vi "list and create PG table 64.vi"(6 "columns type (real)":string="real", 8 "error in":errorcluster, 9 "columns":string[](array[string]), 10 "table name":string, 11 "conn":u64) -> (0 "error out":errorcluster, 3 "conn_out":u64)   [LabVIEW 2019, in "PostgreSQL.lvlib"]
uses:
  PostgreSQL.lvlib
  PostgreSQL2LabVIEW/libpqlv64/src/PQresultErrorMessage.vi
  PostgreSQL2LabVIEW/libpqUtility64/src/PQclear.vi
  PostgreSQL2LabVIEW/libpqlv64/src/PQsendQuery.vi
  PostgreSQL2LabVIEW/libpqlv64/src/PQgetResult.vi
  PostgreSQL2LabVIEW/libpqlv64/src/PQresultStatus.vi
  PostgreSQL2LabVIEW/libpqUtility64/src/PQgetColumn.vi
  PostgreSQL2LabVIEW/libpqlv64/src/PQclear.vi
  PostgreSQL2LabVIEW/libpqUtility64/src/PQfetchTables.vi
  PostgreSQL2LabVIEW/libpqlv64/src/PQgetvalue.vi
  PostgreSQL2LabVIEW/libpqlv64/src/PQntuples.vi
  PostgreSQL2LabVIEW/libpqUtility64/libpqutility64.lvlib
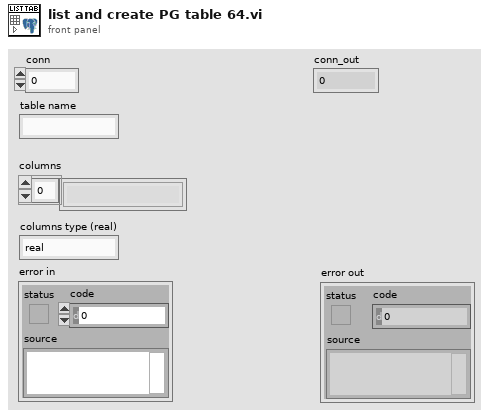
[diagram p1: front panel]
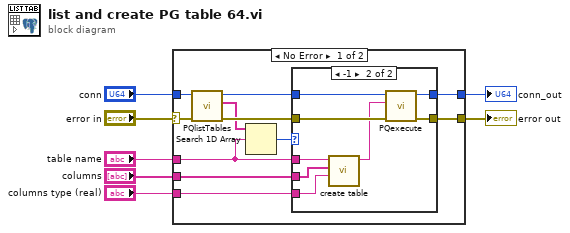
[diagram p0: block diagram]
diagram:
  n1 = case shown="No Error" "error in" {
    selector: "error in" -> [w16 w30]
    tunnel: "conn" -> [w13 w29]
    tunnel: [w18 w29] -> w5
    tunnel: "columns" -> [w12 _]
    tunnel: [w17 w30] -> w4
    tunnel: "table name" -> [w9 _]
    tunnel: "columns type (real)" -> [w11 _]
    frame No Error {
      n2 = call "PQlistTables.vi"("error in"=w16, "conn"=w13) -> ("error out"=w15:errorcluster, "Data"=w10:string[], "conn_out"=w14:u64)  [unwired: 7 in]
      n3 = Search 1D Array(1D array=w10, element=w9) -> (index of element=w8:i32)  [unwired: 1 in]
      n4 = case shown="-1" w8 {
        tunnel: w14 -> [w20 w26]
        tunnel: [w20 w24] -> w18
        tunnel: w15 -> [w19 w25]
        tunnel: [w19 w23] -> w17
        tunnel: w12 -> [_ w27]
        tunnel: w9 -> [_ w28]
        tunnel: w11 -> [_ w22]
        frame 0, Default {
        }
        frame -1 {
          n5 = call "create table.vi"("columns type (real)"=w22, "columns"=w27, "table name"=w28) -> ("create table parameters"=w21:string)  [unwired: 8 in]
          n6 = call "PQexecute.vi"("error in"=w25, "SQL querry"=w21, "conn"=w26) -> ("error out"=w23:errorcluster, "conn_out"=w24:u64)  [unwired: 7 in]
        }
      }
    }
    frame Error {
    }
  }
  "conn_out" <- w5
  "error out" <- w4
